vi "sub_waypoint_math.vi"(9 "lookahead distance":dbl, 10 "waypoint out":cluster{"x":dbl, "y":dbl}[](array[cluster]), 11 "tm out":cluster{dbl, dbl}) -> (3 "waypoint analysis format":T1)   [LabVIEW 2019]
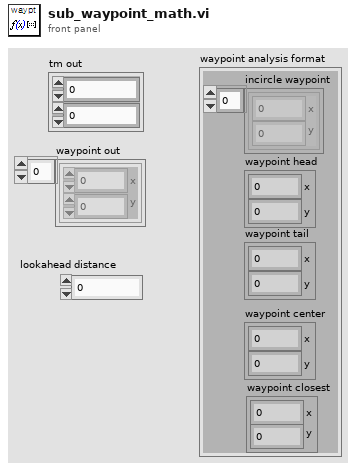
[diagram p1: front panel]
types:
  T1 = cluster{"incircle waypoint":cluster{"x":dbl, "y":dbl}[], "waypoint head":cluster{"x":dbl, "y":dbl}, "waypoint tail":cluster{"x":dbl, "y":dbl}, "waypoint center":cluster{"x":dbl, "y":dbl}, "waypoint closest":cluster{"x":dbl, "y":dbl}}
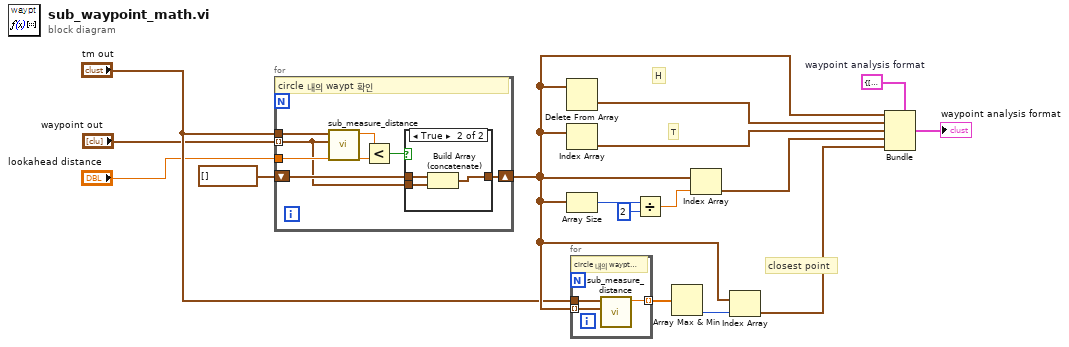
[diagram p0: block diagram]
diagram:
  w15 = T1 {"incircle waypoint"=[], "waypoint head"={"x"=0.0, "y"=0.0}, "waypoint tail"={"x"=0.0, "y"=0.0}, "waypoint center"={"x"=0.0, "y"=0.0}, "waypoint closest"={"x"=0.0, "y"=0.0}}  # waypoint analysis format
  # "closest point"
  # "T"
  # "H"
  n1 = for {
    tunnel: "waypoint out" -> [w18] mode=indexing
    tunnel: "tm out" -> [w23]
    shift-right: [w17] -> w13
    shift-left: cluster{"x":dbl, "y":dbl}[] [] -> [w20]
    tunnel: "lookahead distance" -> [w21]
    # "circle 내의 waypt 확인"
    n2 = call "sub_measure_distance.vi"("pt 2"=w18, "pt 1"=w23) -> ("distance"=w22:dbl)  [unwired: 9 in]
    n3 = Less?(x=w22, y=w21) -> (x < y?=w19:bool)
    n4 = case shown="True" w19 {
      tunnel: w20 -> [w24 w27]
      tunnel: w18 -> [_ w26]
      tunnel: [w24 w25] -> w17
      frame False {
      }
      frame True {
        n5 = Build Array (concatenate)(w27, w26) -> (w25:cluster{"x":dbl, "y":dbl}[])
      }
    }
  }
  n6 = Delete From Array(array=w13) -> (deleted portion=w7:cluster{"x":dbl, "y":dbl})  [unwired: 2 in, 1 out]
  n7 = Index Array(array=w13) -> (element=w8:cluster{"x":dbl, "y":dbl})  [unwired: 1 in]
  n8 = Array Size(array=w13) -> (size(s)=w4:i32)
  n9 = for {
    tunnel: w13 -> [w29] mode=indexing
    tunnel: "tm out" -> [w30]
    tunnel: [w28] -> w10 mode=indexing
    # "circle 내의 waypt 확인"
    n10 = call "sub_measure_distance.vi"("pt 2"=w29, "pt 1"=w30) -> ("distance"=w28:dbl)  [unwired: 9 in]
  }
  n11 = Divide(x=w4, y=2) -> (x/y=w6:dbl)
  n12 = Array Max & Min(array=w10) -> (min index (indices)=w11:i32)  [unwired: 3 out]
  n13 = Index Array(array=w13, index=w6) -> (element=w9:cluster{"x":dbl, "y":dbl})
  n14 = Index Array(array=w13, index=w11) -> (element=w14:cluster{"x":dbl, "y":dbl})
  n15 = Bundle(cluster=w15, "incircle waypoint"=w13, "waypoint head"=w7, "waypoint tail"=w8, "waypoint center"=w9, "waypoint closest"=w14) -> (→"waypoint analysis format":T1)
